vi "HandleAttract.vi"(8 "error in (no error)":errorcluster, 10 "AnyKey?":bool, 11 "Engine in":refnum<class "Engine.lvclass">) -> (0 "error out":errorcluster, 3 "Engine out":refnum<class "Engine.lvclass">)   [LabVIEW 2019, in "RT_Game.lvlib" / "Engine.lvclass"]
uses:
  Engine.lvclass
  Engine.lvclass/Engine.ctl
  Globals.vi
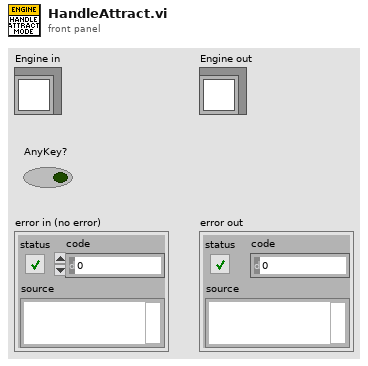
[diagram p1: front panel]
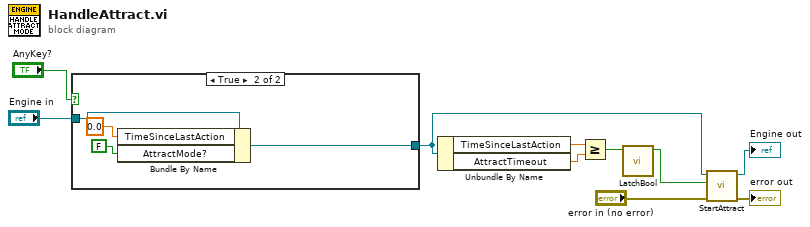
[diagram p0: block diagram]
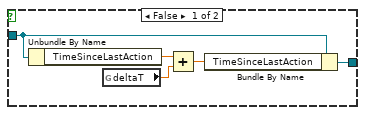
[diagram p2: hidden frame]
diagram:
  n1 = case shown="True" "AnyKey?" {
    tunnel: "Engine in" -> [w14 w19]
    tunnel: [w15 w18] -> w2
    frame False {
      n2 = Unbundle By Name(w14) -> ("TimeSinceLastAction"=w13:dbl)
      n3 = global read "Globals.vi" "deltaT"() -> (w12:dbl)
      n4 = Add(x=w13, y=w12) -> (x+y=w11:dbl)
      n5 = Bundle By Name(cluster=w14, "TimeSinceLastAction"=w11) -> (w15:refnum<class "Engine.lvclass">)
    }
    frame True {
      n6 = Bundle By Name(cluster=w19, "TimeSinceLastAction"=0.0, "AttractMode?"=FALSE) -> (w18:refnum<class "Engine.lvclass">)
    }
  }
  n7 = Unbundle By Name(w2) -> ("TimeSinceLastAction"=w7:dbl, "AttractTimeout"=w6:dbl)
  n8 = Greater Or Equal?(x=w7, y=w6) -> (x >= y?=w5:bool)
  n9 = call "LatchBool.vi"("Boolean"=w5) -> ("Latched Boolean"=w1:bool)  [unwired: 10 in]
  n10 = call "StartAttract.vi"("error in (no error)"="error in (no error)", "Start?"=w1, "Engine in"=w2) -> ("error out"=→"error out":errorcluster, "Engine out"=→"Engine out":refnum<class "Engine.lvclass">)  [unwired: 7 in]
